vi "CALC_Bridge_and_clamp_swap_(arr).vi"(9 "Twisted neck":bool, 10 "Bridge swap":bool, 11 "Data array in":T1[](array[typedef])) -> (3 "Data array out":T1[](array[typedef]))   [LabVIEW 2018, in "Tracker.lvlib"]
uses:
  Tracker.lvlib
  Controls/CTL_Animal_Coordinates_and_Speed.ctl
  Common_Resources.lvlib
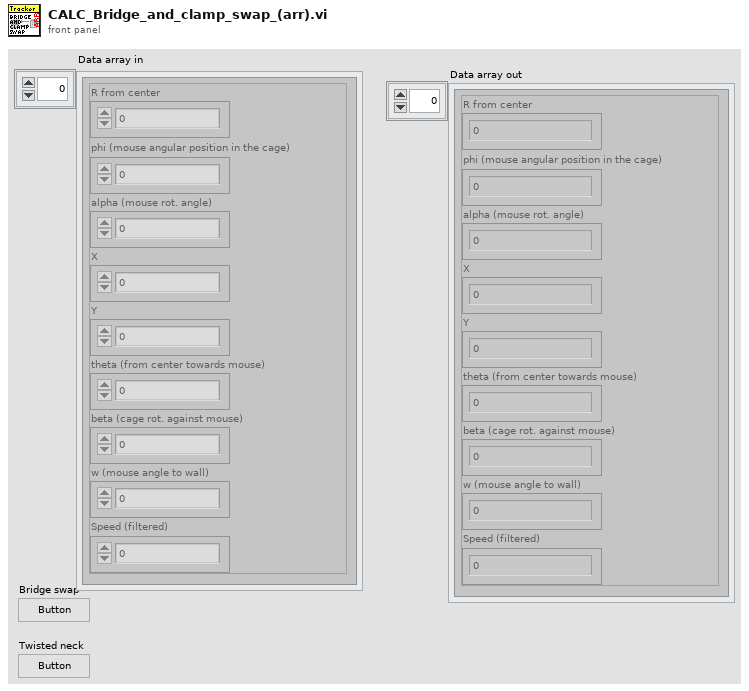
[diagram p1: front panel]
types:
  T1 = typedef "Common_Resources.lvlib/CTL_Animal_Coordinates_and_Speed.ctl" = cluster{"R from center":dbl, "phi (mouse angular position in the cage)":dbl, "alpha (mouse rot. angle)":dbl, "X":dbl, "Y":dbl, "theta (from center towards mouse)":dbl, "beta (cage rot. against mouse)":dbl, "w (mouse angle to wall)":dbl, "Speed (filtered)":dbl}
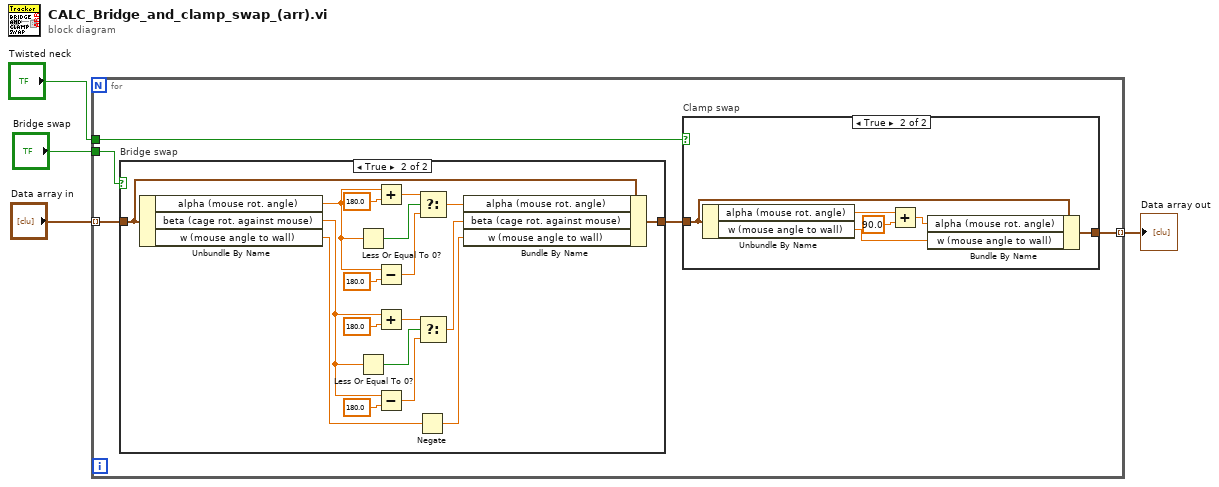
[diagram p0: block diagram]
diagram:
  n1 = for {
    tunnel: "Twisted neck" -> [w9]
    tunnel: "Bridge swap" -> [w5]
    tunnel: "Data array in" -> [w6] mode=indexing
    tunnel: [w8] -> w1 mode=indexing
    n2 = case "Bridge swap" shown="True" w5 {
      tunnel: [w17 w29] -> w7
      tunnel: w6 -> [w17 w30]
      frame False {
      }
      frame True {
        n3 = Unbundle By Name(w30) -> ("alpha (mouse rot. angle)"=w28:dbl, "beta (cage rot. against mouse)"=w21:dbl, "w (mouse angle to wall)"=w19:dbl)
        n4 = Less Or Equal To 0?(x=w28) -> (x <= 0?=w35:bool)
        n5 = Less Or Equal To 0?(x=w21) -> (x <= 0?=w22:bool)
        n6 = Add(x=w28, y=sgl 180.0) -> (x+y=w32:dbl)
        n7 = Subtract(x=w28, y=sgl 180.0) -> (x-y=w34:dbl)
        n8 = Add(x=w21, y=sgl 180.0) -> (x+y=w25:dbl)
        n9 = Subtract(x=w21, y=sgl 180.0) -> (x-y=w23:dbl)
        n10 = Negate(x=w19) -> (-x=w18:dbl)
        n11 = Select(t=w32, s=w35, f=w34) -> (s? t:f=w27:dbl)
        n12 = Select(t=w25, s=w22, f=w23) -> (s? t:f=w20:dbl)
        n13 = Bundle By Name(cluster=w30, "alpha (mouse rot. angle)"=w27, "beta (cage rot. against mouse)"=w20, "w (mouse angle to wall)"=w18) -> (w29:T1)
      }
    }
    n14 = case "Clamp swap" shown="True" w9 {
      tunnel: [w10 w14] -> w8
      tunnel: w7 -> [w10 w15]
      frame False {
      }
      frame True {
        n15 = Unbundle By Name(w15) -> ("alpha (mouse rot. angle)"=w13:dbl, "w (mouse angle to wall)"=w12:dbl)
        n16 = Add(x=w13, y=sgl 90.0) -> (x+y=w11:dbl)
        n17 = Bundle By Name(cluster=w15, "alpha (mouse rot. angle)"=w11, "w (mouse angle to wall)"=w12) -> (w14:T1)
      }
    }
  }
  "Data array out" <- w1
